vi "Write Private Info.vi"(6 "Info":string, 11 "Executioner in":refnum<class "Executioner.lvclass">) -> (3 "Executioner out":refnum<class "Executioner.lvclass">)   [LabVIEW 2017, in "Test Executive.lvlib" / "Executioner.lvclass"]
uses:
  <vilib>/gpm_packages/@cs/test-executive/Source/Test Executive/Executioner/Executioner.lvclass
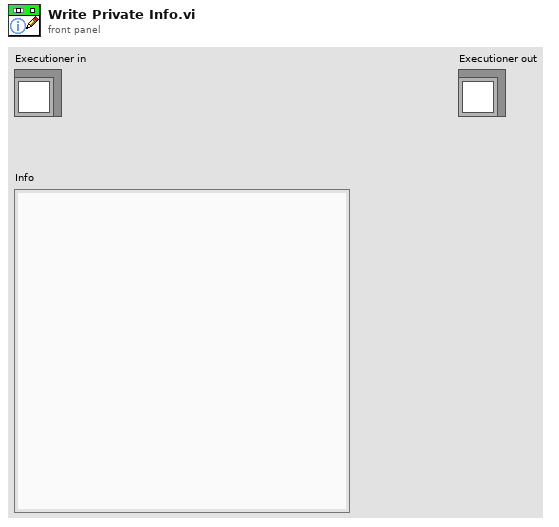
[diagram p1: front panel]
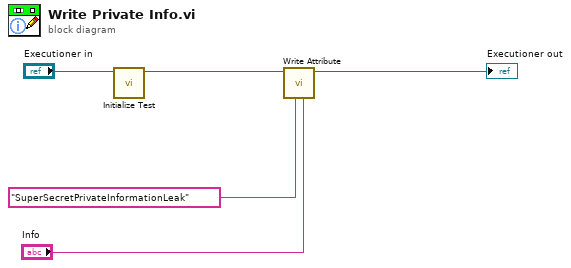
[diagram p0: block diagram]
diagram:
  n1 = call <vilib>:"Initialize Test.vi"("Executioner in"="Executioner in") -> ("Executioner out"=w1:refnum<class "Executioner.lvclass">)  [unwired: 10 in]
  n2 = call <vilib>:"Write Attribute.vi"("Attribute"="Info", "Attribute Name"="SuperSecretPrivateInformationLeak", "Executioner in"=w1) -> ("Executioner out"=→"Executioner out":refnum<class "Executioner.lvclass">)  [unwired: 8 in]
